vi "Take Measurement.vi"(4 "stop?":bool, 6 "initialize?":bool, 8 "error in (no error)":errorcluster, 10 "Transport in":refnum<class "SMO.Transport.lvclass">, 11 "SweepControl in":refnum<class "SMO.SweepControl.lvclass">) -> (0 "error out":errorcluster, 1 "Control Experiment.lvclass":refnum<class "Control Experiment.lvclass">, 2 "Transport out":refnum<class "SMO.Transport.lvclass">, 3 "SweepControl":refnum<class "SMO.SweepControl.lvclass">)   [LabVIEW 2019, in "SMO.SweepControl.lvclass"]
uses:
  SMO.SweepControl.lvclass
  SMO.Transport/SMO.Transport.lvclass
  Control Experiment/Control Experiment.lvclass
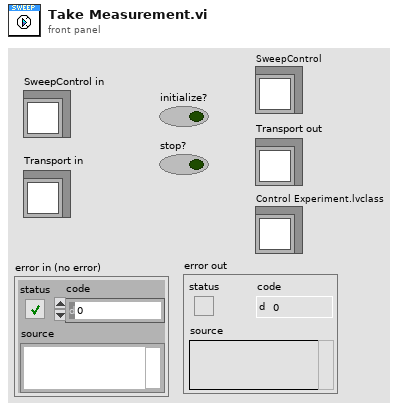
[diagram p1: front panel]
types:
  T1 = typedef "SMO.Transport.lvclass/Dependencies--Cluster.ctl" = cluster{"Control Experiment":refnum<class "Control Experiment.lvclass">}
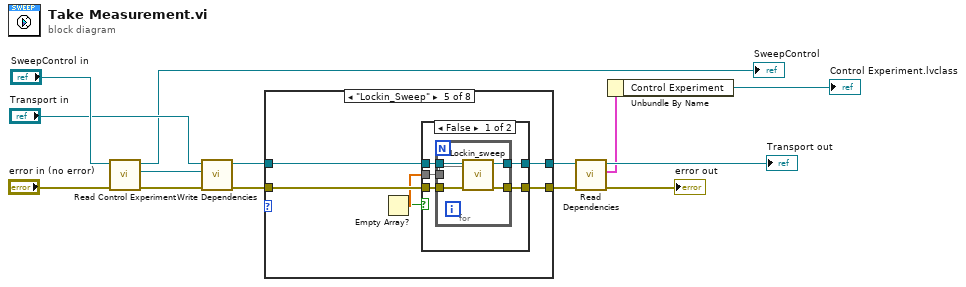
[diagram p0: block diagram]
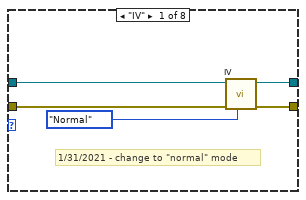
[diagram p2: hidden frame]
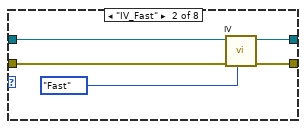
[diagram p3: hidden frame]
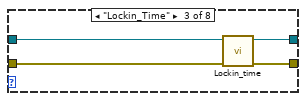
[diagram p4: hidden frame]
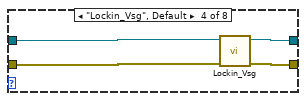
[diagram p5: hidden frame]
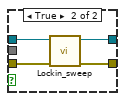
[diagram p6: hidden frame]
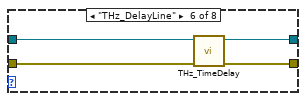
[diagram p7: hidden frame]
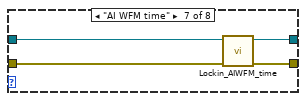
[diagram p8: hidden frame]
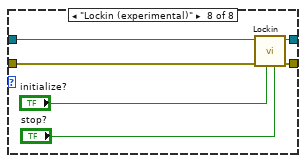
[diagram p9: hidden frame]
diagram:
  n1 = call "Read Control Experiment.vi"("error in (no error)"="error in (no error)", "SweepControl in"="SweepControl in") -> ("error out"=w11:errorcluster, "Control Experiment.lvclass"=w1:refnum<class "Control Experiment.lvclass">, "SweepControl out"=→"SweepControl":refnum<class "SMO.SweepControl.lvclass">)  [unwired: 7 in]
  n2 = call "Write Dependencies.vi"("error in (no error)"=w11, "Control Experiment.lvclass"=w1, "Transport in"="Transport in") -> ("error out"=w15:errorcluster, "Transport out"=w14:refnum<class "SMO.Transport.lvclass">)  [unwired: 7 in]
  n3 = case shown="\"Lockin_Sweep\"" w13 {
    tunnel: w15 -> [w20 w25 w29 w33 w39 w57 w61 w67]
    tunnel: w14 -> [w19 w24 w28 w32 w38 w56 w60 w66]
    tunnel: [w18 w23 w27 w31 w37 w55 w59 w65] -> w7
    tunnel: [w16 w21 w26 w30 w36 w54 w58 w62] -> w6
    frame "IV" {
      # "1/31/2021 - change to \"normal\" mode"
      n4 = call "IV.vi"("Speed"=enum16{"Normal", "Fast", "Instant"}."Normal", "error in"=w20, "Transport"=w19) -> ("error out"=w18:errorcluster, "Transport out"=w16:refnum<class "SMO.Transport.lvclass">)  [unwired: 7 in]
    }
    frame "IV_Fast" {
      n5 = call "IV.vi"("Speed"=enum16{"Normal", "Fast", "Instant"}."Fast", "error in"=w25, "Transport"=w24) -> ("error out"=w23:errorcluster, "Transport out"=w21:refnum<class "SMO.Transport.lvclass">)  [unwired: 7 in]
    }
    frame "Lockin_Time" {
      n6 = call "Lockin_time.vi"("error in (no error)"=w29, "Transport"=w28) -> ("error out"=w27:errorcluster, "Transport out"=w26:refnum<class "SMO.Transport.lvclass">)  [unwired: 8 in]
    }
    frame "Lockin_Vsg", Default {
      n7 = call "Lockin_Vsg.vi"("error in (no error)"=w33, "Transport"=w32) -> ("error out"=w31:errorcluster, "Transport out"=w30:refnum<class "SMO.Transport.lvclass">)  [unwired: 8 in]
    }
    frame "Lockin_Sweep" {
      n8 = Empty Array?() -> (array=w35:ext[], empty?=w34:bool)
      n9 = case shown="False" w34 {
        tunnel: w39 -> [w44 w53]
        tunnel: w38 -> [w43 w52]
        tunnel: [w42 w51] -> w37
        tunnel: [w41 w50] -> w36
        tunnel: w35 -> [w40 _]
        frame False {
          n10 = for {
            tunnel: w43 -> [w48]
            tunnel: [w46] -> w41
            tunnel: w44 -> [w49]
            tunnel: [w47] -> w42
            tunnel: w40 -> [w45]
            n11 = call "Lockin_sweep.vi"("error in (no error)"=w49, "Configure Sweep"=w45, "Transport"=w48) -> ("error out"=w47:errorcluster, "Transport out"=w46:refnum<class "SMO.Transport.lvclass">)  [unwired: 7 in]
          }
        }
        frame True {
          n12 = call "Lockin_sweep.vi"("error in (no error)"=w53, "Transport"=w52) -> ("error out"=w51:errorcluster, "Transport out"=w50:refnum<class "SMO.Transport.lvclass">)  [unwired: 8 in]
        }
      }
    }
    frame "THz_DelayLine" {
      n13 = call "THz_TimeDelay.vi"("error in (no error)"=w57, "Transport"=w56) -> ("error out"=w55:errorcluster, "Transport out"=w54:refnum<class "SMO.Transport.lvclass">)  [unwired: 8 in]
    }
    frame "AI WFM time" {
      n14 = call "Lockin_AIWFM_time.vi"("error in (no error)"=w61, "Transport"=w60) -> ("error out"=w59:errorcluster, "Transport out"=w58:refnum<class "SMO.Transport.lvclass">)  [unwired: 8 in]
    }
    frame "Lockin (experimental)" {
      n15 = call "Lockin.vi"("stop?"="stop?", "initialize?"="initialize?", "error in (no error)"=w67, "Transport"=w66) -> ("error out"=w65:errorcluster, "Transport out"=w62:refnum<class "SMO.Transport.lvclass">)  [unwired: 6 in]
    }
  }
  n16 = call "Read Dependencies.vi"("error in (no error)"=w7, "Transport in"=w6) -> ("error out"=→"error out":errorcluster, "Dependencies"=w4:T1, "Transport out"=→"Transport out":refnum<class "SMO.Transport.lvclass">)  [unwired: 7 in]
  n17 = Unbundle By Name(w4) -> ("Control Experiment"=→"Control Experiment.lvclass":refnum<class "Control Experiment.lvclass">)
